vi "TwoBallAuton.vi"(11 "Intake Suck at Beginning?":bool) -> ()   [LabVIEW 2013]
uses:
  <vilib>/Rock Robotics/WPI/SafetyOutput/WPI_SafetyOutputConfigMenu.ctl
  <vilib>/Rock Robotics/WPI/Solenoid/WPI_SolenoidValue.ctl
  <vilib>/Rock Robotics/WPI/RobotDrive/WPI_RobotDriveGetSetRefNum.vi
  <vilib>/Rock Robotics/WPI/Solenoid/WPI_SolenoidSetEnum.vi
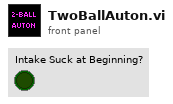
[diagram p1: front panel]
types:
  T1 = typedef "WPI_SafetyOutputConfigMenu.ctl" = enum16{"Enable", "Disable"}
  T2 = typedef "WPI_RobotDriveDevRef.ctl" = cluster{"DevStatus":errorcluster, "Motors[]":T3[], "Square Inputs":bool, "Max Output":dbl, "Isochronous":bool}
  T3 = typedef "WPI_MotorControlDeviceRef.ctl" = cluster{"DeviceStatus":errorcluster, "Type":enum16{"PWM", "CAN"}, "PWM":cluster{"Digital Module":T4, "PWM Channel":T5, "DeadBand":T6}, "CAN":cluster{"Device Number":u8, "Control Mode":T7, "Semaphore":T8, "Max Vout":dbl}, "Invert":bool, "TransformRef":T9, "InvTransformRef":T9}
  T4 = typedef "FPGA_TypedefDigitalModule.ctl" = enum16{"Digital Module 1", "Digital Module 2"}
  T5 = typedef "FPGA_DIOPWMChannel.ctl" = enum8{"PWM 1", "PWM 2", "PWM 3", "PWM 4", "PWM 5", "PWM 6", "PWM 7", "PWM 8", "PWM 9", "PWM 10", "Invalid"}
  T6 = typedef "WPI_PWMDeadband.ctl" = cluster{"Name":string, "maxPositivePwm":i32, "minPositivePwm":i32, "centerPwm":i32, "maxNegativePwm":i32, "minNegativePwm":i32, "angularRange":u16}
  T7 = typedef "WPI_CANJaguar_ControlMode.ctl" = enum8{"Percent VBus", "Current", "Speed", "Position", "Voltage"}
  T8 = typedef "Semaphore RefNum" = refnum<k1>
  T9 = typedef "WPI_PWMTransform_ConPane.ctl" = refnum<vi>
  T10 = typedef "WPI_DigitalInputDevRef.ctl" = cluster{"DevStatus":errorcluster, "DIO Channel":T11, "Digital Module":T4}
  T11 = typedef "FPGA_DIOChannel.ctl" = enum8{"DIO 1", "DIO 2", "DIO 3", "DIO 4", "DIO 5", "DIO 6", "DIO 7", "DIO 8", "DIO 9", "DIO 10", "DIO 11", "DIO 12", "DIO 13", "DIO 14", "Invalid"}
  T12 = typedef "WPI_SolenoidDevRef.ctl" = cluster{"DevStatus":errorcluster, "Solenoid Module":T13, "Forward Solenoid Channel":T14, "Reverse Solenoid Channel":T14}
  T13 = typedef "FPGA_TypedefSolenoidModule.ctl" = enum16{"Solenoid Module 1", "Solenoid Module 2"}
  T14 = typedef "WPI_SolenoidChannel.ctl" = enum8{"Solenoid 1", "Solenoid 2", "Solenoid 3", "Solenoid 4", "Solenoid 5", "Solenoid 6", "Solenoid 7", "Solenoid 8", "Invalid"}
  T15 = typedef "WPI_EncoderDevRef.ctl" = cluster{"DevStatus":errorcluster, "EncoderIndex":T16, "CounterIndex":T17, "DistancePerCount":dbl, "Decoding Type":T18}
  T16 = typedef "FPGA_EncoderIdx.ctl" = enum8{"Enc 0", "Enc 1", "Enc 2", "Enc 3", "Invalid"}
  T17 = typedef "FPGA_CounterCtrSystemIndex.ctl" = enum8{"Ctr 0", "Ctr 1", "Ctr 2", "Ctr 3", "Ctr 4", "Ctr 5", "Ctr 6", "Ctr 7", "Invalid"}
  T18 = typedef "WPI_EncoderType.ctl" = enum16{"1x", "2x", "4x"}
  T19 = typedef "WPI_SolenoidValue.ctl" = enum16{"Off", "On", "Forward", "Reverse"}
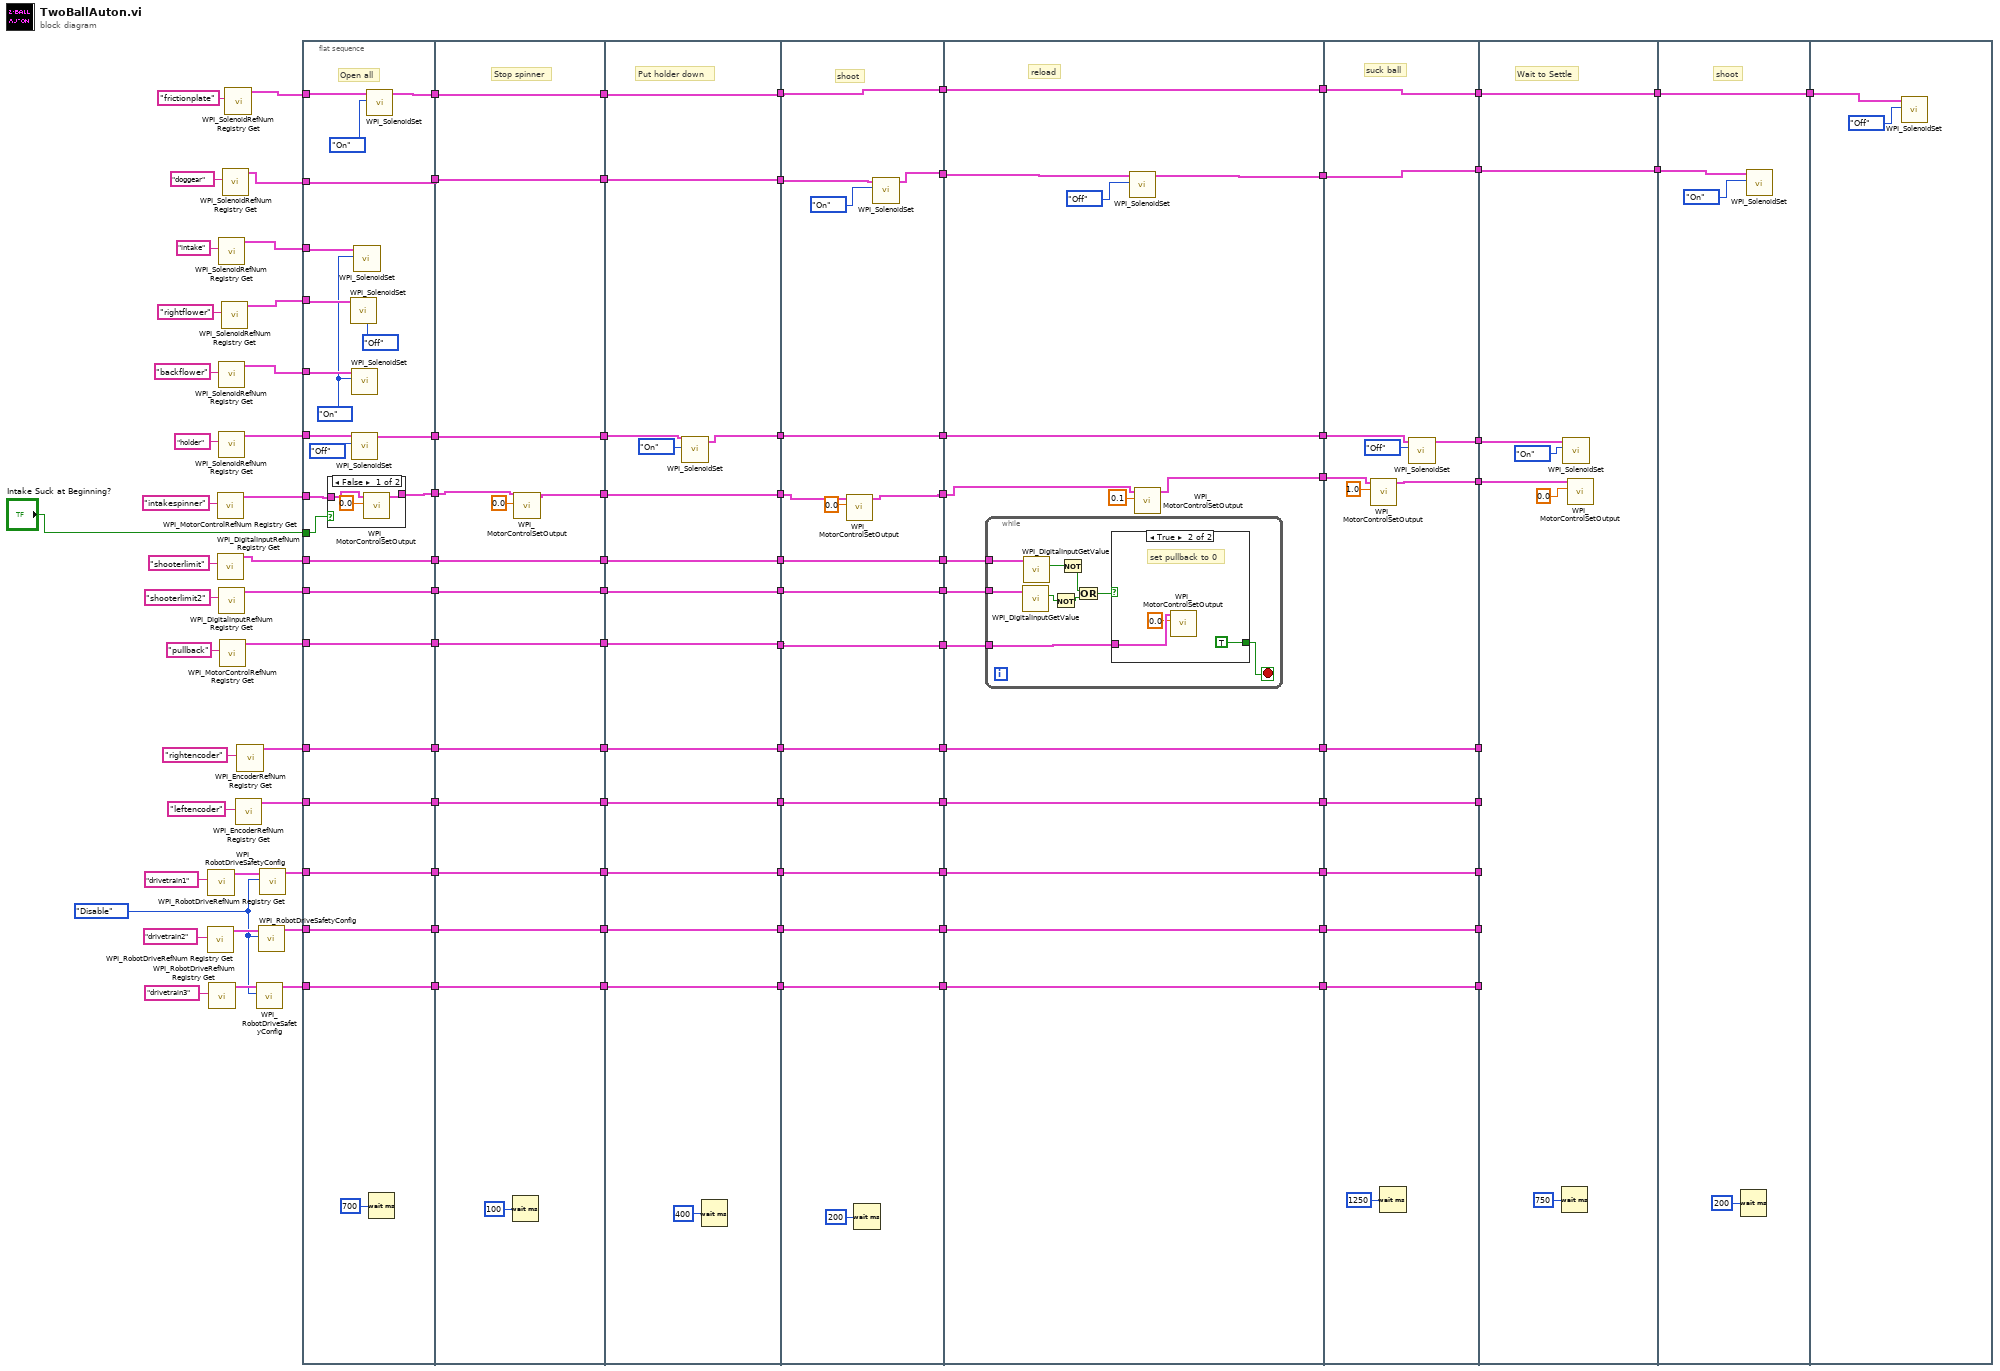
[diagram p0: block diagram]
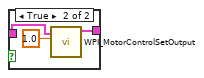
[diagram p2: hidden frame]
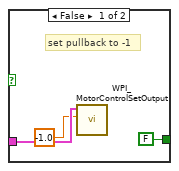
[diagram p3: hidden frame]
diagram:
  w51 = WPI_SafetyOutputConfigMenu."Disable" ("mode")
  n1 = call <vilib>:"WPI_RobotDriveRefNum Registry Get.vi"("refnum name"="drivetrain2") -> ("RobotDriveDevRef"=w53:T2)  [unwired: 9 in, 1 out]
  n2 = call <vilib>:"WPI_RobotDriveRefNum Registry Get.vi"("refnum name"="drivetrain1") -> ("RobotDriveDevRef"=w54:T2)  [unwired: 9 in, 1 out]
  n3 = call <vilib>:"WPI_RobotDriveRefNum Registry Get.vi"("refnum name"="drivetrain3") -> ("RobotDriveDevRef"=w52:T2)  [unwired: 9 in, 1 out]
  n4 = call <vilib>:"WPI_MotorControlRefNum Registry Get.vi"("refnum name"="intakespinner") -> ("MotorControlDevRef"=w64:T3)  [unwired: 9 in, 1 out]
  n5 = call <vilib>:"WPI_DigitalInputRefNum Registry Get.vi"("refnum name"="shooterlimit") -> ("DigitalInputDevRef"=w62:T10)  [unwired: 9 in, 1 out]
  n6 = call <vilib>:"WPI_SolenoidRefNum Registry Get.vi"("refnum name"="intake") -> ("SolenoidDevRef"=w68:T12)  [unwired: 9 in, 1 out]
  n7 = call <vilib>:"WPI_SolenoidRefNum Registry Get.vi"("refnum name"="backflower") -> ("SolenoidDevRef"=w66:T12)  [unwired: 9 in, 1 out]
  n8 = call <vilib>:"WPI_SolenoidRefNum Registry Get.vi"("refnum name"="holder") -> ("SolenoidDevRef"=w32:T12)  [unwired: 9 in, 1 out]
  n9 = call <vilib>:"WPI_DigitalInputRefNum Registry Get.vi"("refnum name"="shooterlimit2") -> ("DigitalInputDevRef"=w36:T10)  [unwired: 9 in, 1 out]
  n10 = call <vilib>:"WPI_MotorControlRefNum Registry Get.vi"("refnum name"="pullback") -> ("MotorControlDevRef"=w60:T3)  [unwired: 9 in, 1 out]
  n11 = call <vilib>:"WPI_SolenoidRefNum Registry Get.vi"("refnum name"="rightflower") -> ("SolenoidDevRef"=w67:T12)  [unwired: 9 in, 1 out]
  n12 = call <vilib>:"WPI_SolenoidRefNum Registry Get.vi"("refnum name"="doggear") -> ("SolenoidDevRef"=w72:T12)  [unwired: 9 in, 1 out]
  n13 = call <vilib>:"WPI_SolenoidRefNum Registry Get.vi"("refnum name"="frictionplate") -> ("SolenoidDevRef"=w43:T12)  [unwired: 9 in, 1 out]
  n14 = call <vilib>:"WPI_EncoderRefNum Registry Get.vi"("refnum name"="leftencoder") -> ("EncoderDevRef"=w49:T15)  [unwired: 9 in, 1 out]
  n15 = call <vilib>:"WPI_EncoderRefNum Registry Get.vi"("refnum name"="rightencoder") -> ("EncoderDevRef"=w50:T15)  [unwired: 9 in, 1 out]
  n16 = call <vilib>:"WPI_RobotDriveSafetyConfig.vi"("mode"=w51, "RobotDriveDevRef"=w52) -> ("RobotDriveDevRef"=w46:T2)  [unwired: 8 in, 1 out]
  n17 = call <vilib>:"WPI_RobotDriveSafetyConfig.vi"("mode"=w51, "RobotDriveDevRef"=w53) -> ("RobotDriveDevRef"=w47:T2)  [unwired: 8 in, 1 out]
  n18 = call <vilib>:"WPI_RobotDriveSafetyConfig.vi"("mode"=w51, "RobotDriveDevRef"=w54) -> ("RobotDriveDevRef"=w48:T2)  [unwired: 8 in, 1 out]
  n19 = flat-sequence {
    tunnel: w72 -> [w128]
    tunnel: [w128] -> w27
    tunnel: w68 -> [w127]
    tunnel: w67 -> [w126]
    tunnel: w66 -> [w125]
    tunnel: w64 -> [w123]
    tunnel: [w122] -> w26
    tunnel: w62 -> [w121]
    tunnel: [w121] -> w25
    tunnel: w60 -> [w120]
    tunnel: [w120] -> w24
    tunnel: [w119] -> w23
    tunnel: w50 -> [w119]
    tunnel: [w118] -> w22
    tunnel: w49 -> [w118]
    tunnel: [w117] -> w21
    tunnel: w48 -> [w117]
    tunnel: [w116] -> w20
    tunnel: w47 -> [w116]
    tunnel: [w115] -> w19
    tunnel: w46 -> [w115]
    tunnel: "Intake Suck at Beginning?" -> [w112]
    tunnel: w43 -> [w110]
    tunnel: [w109] -> w18
    tunnel: w36 -> [w108]
    tunnel: [w108] -> w17
    tunnel: w32 -> [w107]
    tunnel: [w105] -> w16
    tunnel: w27 -> [w149]
    tunnel: [w149] -> w15
    tunnel: w26 -> [w137]
    tunnel: w25 -> [w148]
    tunnel: [w148] -> w14
    tunnel: w24 -> [w147]
    tunnel: [w147] -> w13
    tunnel: w23 -> [w146]
    tunnel: [w146] -> w12
    tunnel: w22 -> [w145]
    tunnel: [w145] -> w11
    tunnel: w21 -> [w144]
    tunnel: [w144] -> w10
    tunnel: w20 -> [w143]
    tunnel: [w143] -> w9
    tunnel: w19 -> [w142]
    tunnel: [w142] -> w8
    tunnel: w18 -> [w141]
    tunnel: [w141] -> w7
    tunnel: w17 -> [w140]
    tunnel: [w140] -> w6
    tunnel: w16 -> [w139]
    tunnel: [w139] -> w5
    tunnel: [w136] -> w4
    tunnel: [w151] -> w104
    tunnel: [w163] -> w103
    tunnel: [w162] -> w102
    tunnel: [w161] -> w101
    tunnel: [w160] -> w100
    tunnel: [w159] -> w99
    tunnel: [w158] -> w98
    tunnel: [w157] -> w97
    tunnel: [w156] -> w96
    tunnel: [w155] -> w40
    tunnel: [w154] -> w35
    tunnel: [w152] -> w31
    tunnel: w15 -> [w161]
    tunnel: w14 -> [w163]
    tunnel: w13 -> [w162]
    tunnel: w12 -> [w159]
    tunnel: w11 -> [w160]
    tunnel: w10 -> [w158]
    tunnel: w9 -> [w157]
    tunnel: w8 -> [w156]
    tunnel: w7 -> [w155]
    tunnel: w6 -> [w154]
    tunnel: w5 -> [w150]
    tunnel: w4 -> [w151]
    tunnel: w104 -> [w179]
    tunnel: [w178] -> w95
    tunnel: w103 -> [w181]
    tunnel: [w181] -> w94
    tunnel: w102 -> [w180]
    tunnel: [w180] -> w93
    tunnel: [w174] -> w92
    tunnel: w101 -> [w173]
    tunnel: [w172] -> w91
    tunnel: w100 -> [w172]
    tunnel: [w171] -> w90
    tunnel: w99 -> [w171]
    tunnel: [w170] -> w89
    tunnel: w98 -> [w170]
    tunnel: [w169] -> w88
    tunnel: w97 -> [w169]
    tunnel: [w168] -> w87
    tunnel: w96 -> [w168]
    tunnel: w40 -> [w167]
    tunnel: [w167] -> w39
    tunnel: w35 -> [w166]
    tunnel: [w166] -> w34
    tunnel: w31 -> [w165]
    tunnel: [w165] -> w30
    tunnel: w95 -> [w183]
    tunnel: w94 -> [w197]
    tunnel: w93 -> [w196]
    tunnel: [w194] -> w86
    tunnel: w92 -> [w193]
    tunnel: [w192] -> w85
    tunnel: w91 -> [w192]
    tunnel: [w191] -> w84
    tunnel: w90 -> [w191]
    tunnel: [w190] -> w83
    tunnel: w89 -> [w190]
    tunnel: [w189] -> w82
    tunnel: w88 -> [w189]
    tunnel: [w188] -> w81
    tunnel: w87 -> [w188]
    tunnel: w39 -> [w187]
    tunnel: [w187] -> w38
    tunnel: w34 -> [w186]
    tunnel: w30 -> [w185]
    tunnel: [w185] -> w29
    tunnel: [w182] -> w1
    tunnel: [w226] -> w74
    tunnel: [w223] -> w75
    tunnel: w86 -> [w226]
    tunnel: w85 -> [w221]
    tunnel: w84 -> [w222]
    tunnel: [w222] -> w76
    tunnel: [w221] -> w77
    tunnel: [w220] -> w78
    tunnel: w83 -> [w220]
    tunnel: [w219] -> w79
    tunnel: w82 -> [w219]
    tunnel: [w218] -> w80
    tunnel: w81 -> [w218]
    tunnel: [w217] -> w42
    tunnel: w38 -> [w217]
    tunnel: w29 -> [w215]
    tunnel: [w214] -> w28
    tunnel: w1 -> [w213]
    tunnel: [w233] -> w3
    tunnel: w80 -> [_]
    tunnel: w79 -> [_]
    tunnel: w78 -> [_]
    tunnel: w77 -> [_]
    tunnel: w76 -> [_]
    tunnel: w75 -> [w230]
    tunnel: w74 -> [w233]
    tunnel: w42 -> [w229]
    tunnel: [w229] -> w2
    tunnel: w28 -> [w228]
    tunnel: [w234] -> w41
    tunnel: w2 -> [w234]
    tunnel: w3 -> [w235]
    tunnel: w41 -> [w238]
    frame #0 {
      w114 = WPI_SolenoidValue."On" ("Value")
      # "Open all"
      n20 = case shown="False" w112 {
        tunnel: w123 -> [w130 w134]
        tunnel: [w129 w132] -> w122
        frame False {
          n21 = call <vilib>:"WPI_MotorControlSetOutput.vi"("Output"=0.0, "MotorControlDevRef"=w130) -> ("MotorControlDevRef"=w129:T3)  [unwired: 7 in, 2 out]
        }
        frame True {
          n22 = call <vilib>:"WPI_MotorControlSetOutput.vi"("Output"=1.0, "MotorControlDevRef"=w134) -> ("MotorControlDevRef"=w132:T3)  [unwired: 7 in, 2 out]
        }
      }
      n23 = call-poly <vilib>:"WPI_SolenoidSet.vi"("Value"=WPI_SolenoidValue."Off", "SolenoidDevRef"=w126) -> ()  [unwired: 8 in, 2 out]
      n24 = call-poly <vilib>:"WPI_SolenoidSet.vi"("Value"=w114, "SolenoidDevRef"=w125) -> ()  [unwired: 8 in, 2 out]
      n25 = call-poly <vilib>:"WPI_SolenoidSet.vi"("Value"=WPI_SolenoidValue."Off", "SolenoidDevRef"=w107) -> ("SolenoidDevRef"=w105:T12)  [unwired: 8 in, 1 out]
      n26 = call-poly <vilib>:"WPI_SolenoidSet.vi"("Value"=w114, "SolenoidDevRef"=w127) -> ()  [unwired: 8 in, 2 out]
      n27 = call-poly <vilib>:"WPI_SolenoidSet.vi"("Value"=WPI_SolenoidValue."On", "SolenoidDevRef"=w110) -> ("SolenoidDevRef"=w109:T12)  [unwired: 8 in, 1 out]
      n28 = Wait (ms)(milliseconds to wait=u32 700) -> ()  [unwired: 1 out]
    }
    frame #1 {
      # "Stop spinner"
      n29 = Wait (ms)(milliseconds to wait=u32 100) -> ()  [unwired: 1 out]
      n30 = call <vilib>:"WPI_MotorControlSetOutput.vi"("Output"=0.0, "MotorControlDevRef"=w137) -> ("MotorControlDevRef"=w136:T3)  [unwired: 7 in, 2 out]
    }
    frame #2 {
      # "Put holder down"
      n31 = call-poly <vilib>:"WPI_SolenoidSet.vi"("Value"=WPI_SolenoidValue."On", "SolenoidDevRef"=w150) -> ("SolenoidDevRef"=w152:T12)  [unwired: 8 in, 1 out]
      n32 = Wait (ms)(milliseconds to wait=u32 400) -> ()  [unwired: 1 out]
    }
    frame #3 {
      # "shoot"
      n33 = call <vilib>:"WPI_MotorControlSetOutput.vi"("Output"=0.0, "MotorControlDevRef"=w179) -> ("MotorControlDevRef"=w178:T3)  [unwired: 7 in, 2 out]
      n34 = Wait (ms)(milliseconds to wait=u32 200) -> ()  [unwired: 1 out]
      n35 = call-poly <vilib>:"WPI_SolenoidSet.vi"("Value"=WPI_SolenoidValue."On", "SolenoidDevRef"=w173) -> ("SolenoidDevRef"=w174:T12)  [unwired: 8 in, 1 out]
    }
    frame #4 {
      # "reload"
      n36 = while {
        tunnel: w197 -> [w206]
        tunnel: w196 -> [w204]
        tunnel: w186 -> [w202]
        stop <- w203 stop-if-true
        n37 = call <vilib>:"WPI_DigitalInputGetValue.vi"("DigitalInputDevRef"=w202) -> ("Value"=w198:bool)  [unwired: 8 in, 2 out]
        n38 = call <vilib>:"WPI_DigitalInputGetValue.vi"("DigitalInputDevRef"=w206) -> ("Value"=w205:bool)  [unwired: 8 in, 2 out]
        n39 = Not(x=w198) -> (.not. x?=w199:bool)
        n40 = Not(x=w205) -> (.not. x?=w201:bool)
        n41 = Or(x=w201, y=w199) -> (x .or. y?=w200:bool)
        n42 = case shown="True" w200 {
          tunnel: w204 -> [w209 w212]
          tunnel: [FALSE TRUE] -> w203
          frame False {
            # "set pullback to -1"
            n43 = call <vilib>:"WPI_MotorControlSetOutput.vi"("Output"=-1.0, "MotorControlDevRef"=w209) -> ()  [unwired: 7 in, 3 out]
          }
          frame True {
            # "set pullback to 0"
            n44 = call <vilib>:"WPI_MotorControlSetOutput.vi"("Output"=0.0, "MotorControlDevRef"=w212) -> ()  [unwired: 7 in, 3 out]
          }
        }
      }
      n45 = call-poly <vilib>:"WPI_SolenoidSet.vi"("Value"=WPI_SolenoidValue."Off", "SolenoidDevRef"=w193) -> ("SolenoidDevRef"=w194:T12)  [unwired: 8 in, 1 out]
      n46 = call <vilib>:"WPI_MotorControlSetOutput.vi"("Output"=0.1, "MotorControlDevRef"=w183) -> ("MotorControlDevRef"=w182:T3)  [unwired: 7 in, 2 out]
    }
    frame #5 {
      # "suck ball"
      n47 = call <vilib>:"WPI_MotorControlSetOutput.vi"("Output"=1.0, "MotorControlDevRef"=w213) -> ("MotorControlDevRef"=w223:T3)  [unwired: 7 in, 2 out]
      n48 = Wait (ms)(milliseconds to wait=u32 1250) -> ()  [unwired: 1 out]
      n49 = call-poly <vilib>:"WPI_SolenoidSet.vi"("Value"=WPI_SolenoidValue."Off", "SolenoidDevRef"=w215) -> ("SolenoidDevRef"=w214:T12)  [unwired: 8 in, 1 out]
    }
    frame #6 {
      # "Wait to Settle"
      n50 = Wait (ms)(milliseconds to wait=u32 750) -> ()  [unwired: 1 out]
      n51 = call-poly <vilib>:"WPI_SolenoidSet.vi"("Value"=WPI_SolenoidValue."On", "SolenoidDevRef"=w228) -> ()  [unwired: 8 in, 2 out]
      n52 = call <vilib>:"WPI_MotorControlSetOutput.vi"("Output"=0.0, "MotorControlDevRef"=w230) -> ()  [unwired: 7 in, 3 out]
    }
    frame #7 {
      # "shoot"
      n53 = Wait (ms)(milliseconds to wait=u32 200) -> ()  [unwired: 1 out]
      n54 = call-poly <vilib>:"WPI_SolenoidSet.vi"("Value"=WPI_SolenoidValue."On", "SolenoidDevRef"=w235) -> ()  [unwired: 8 in, 2 out]
    }
    frame #8 {
      n55 = call-poly <vilib>:"WPI_SolenoidSet.vi"("Value"=WPI_SolenoidValue."Off", "SolenoidDevRef"=w238) -> ()  [unwired: 8 in, 2 out]
    }
  }
